vi "average m_error.vi"(1 "Num lights":dbl=2.0, 2 "Match error":waveform(dbl)[](array[waveform])) -> (0 "avg error":dbl[](array[numeric]))   [LabVIEW 2011]
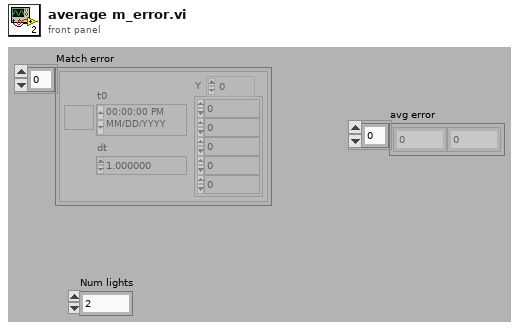
[diagram p1: front panel]
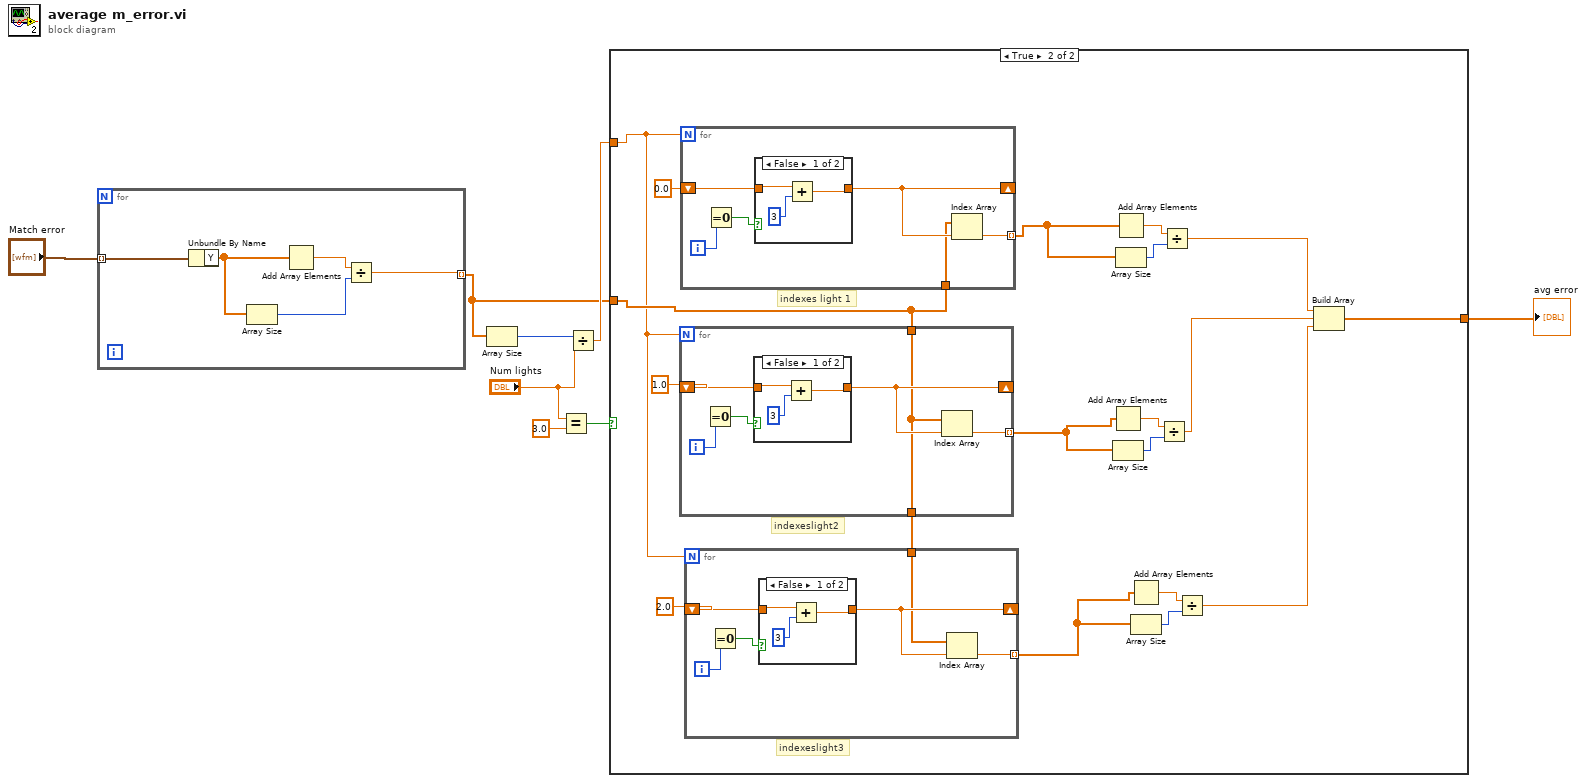
[diagram p0: block diagram]
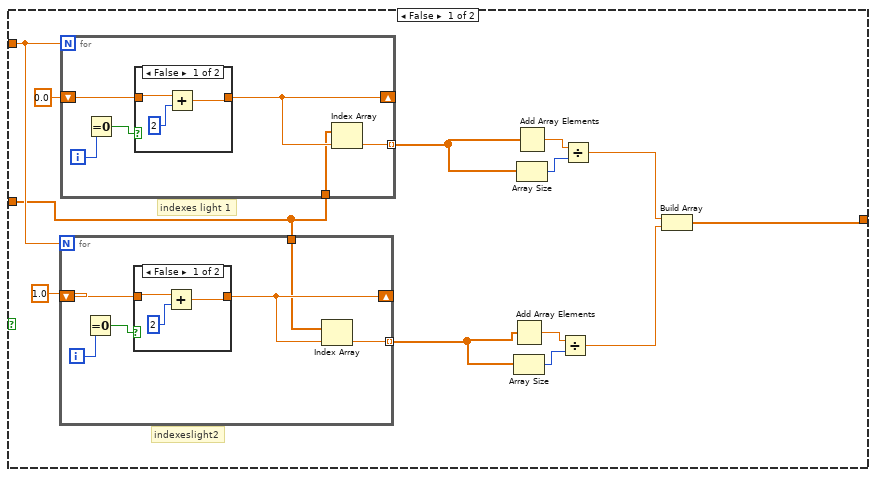
[diagram p2: hidden frame]
diagram:
  n1 = for {
    tunnel: "Match error" -> [w13] mode=indexing
    tunnel: [w9] -> w5 mode=indexing
    n2 = Unbundle By Name(w13) -> ("Y"=w12:dbl[])
    n3 = Array Size(array=w12) -> (size(s)=w10:i32)
    n4 = Add Array Elements(numeric array=w12) -> (sum=w11:dbl)
    n5 = Divide(x=w11, y=w10) -> (x/y=w9:dbl)
  }
  n6 = Array Size(array=w5) -> (size(s)=w7:i32)
  n7 = Equal?(x="Num lights", y=3.0) -> (x = y?=w2:bool)
  n8 = Divide(x=w7, y="Num lights") -> (x/y=w6:dbl)
  n9 = case shown="True" w2 {
    tunnel: w6 -> [w24 w60]
    tunnel: w5 -> [w23 w63]
    tunnel: [w14 w47] -> w1
    frame False {
      # "indexeslight2"
      # "indexes light 1"
      n10 = for {
        N: w24 -> [_]
        shift-right: [w29] -> _
        shift-left: 1.0 -> [w30]
        tunnel: [w28] -> w17 mode=indexing
        tunnel: w23 -> [w27]
        i -> [w32]
        n11 = Equal To 0?(x=w32) -> (x = 0?=w31:bool)
        n12 = case shown="False" w31 {
          tunnel: w30 -> [w35 w36]
          tunnel: [w33 w36] -> w29
          frame False {
            n13 = Add(x=w35, y=2) -> (x+y=w33:dbl)
          }
          frame True {
          }
        }
        n14 = Index Array(array=w27, index=w29) -> (element=w28:dbl)
      }
      n15 = for {
        N: w24 -> [_]
        shift-right: [w39] -> _
        shift-left: 0.0 -> [w40]
        tunnel: [w38] -> w18 mode=indexing
        tunnel: w23 -> [w37]
        i -> [w42]
        n16 = Equal To 0?(x=w42) -> (x = 0?=w41:bool)
        n17 = case shown="False" w41 {
          tunnel: w40 -> [w45 w46]
          tunnel: [w43 w46] -> w39
          frame False {
            n18 = Add(x=w45, y=2) -> (x+y=w43:dbl)
          }
          frame True {
          }
        }
        n19 = Index Array(array=w37, index=w39) -> (element=w38:dbl)
      }
      n20 = Add Array Elements(numeric array=w17) -> (sum=w20:dbl)
      n21 = Array Size(array=w17) -> (size(s)=w19:i32)
      n22 = Add Array Elements(numeric array=w18) -> (sum=w22:dbl)
      n23 = Array Size(array=w18) -> (size(s)=w21:i32)
      n24 = Divide(x=w20, y=w19) -> (x/y=w15:dbl)
      n25 = Divide(x=w22, y=w21) -> (x/y=w16:dbl)
      n26 = Build Array(w16, w15) -> (w14:dbl[])
    }
    frame True {
      # "indexeslight3"
      # "indexeslight2"
      # "indexes light 1"
      n27 = for {
        N: w60 -> [_]
        shift-right: [w78] -> _
        shift-left: 1.0 -> [w79]
        tunnel: [w77] -> w49 mode=indexing
        tunnel: w63 -> [w76]
        tunnel: [w76] -> w61
        i -> [w81]
        n28 = Equal To 0?(x=w81) -> (x = 0?=w80:bool)
        n29 = case shown="False" w80 {
          tunnel: w79 -> [w84 w85]
          tunnel: [w82 w85] -> w78
          frame False {
            n30 = Add(x=w84, y=3) -> (x+y=w82:dbl)
          }
          frame True {
          }
        }
        n31 = Index Array(array=w76, index=w78) -> (element=w77:dbl)
      }
      n32 = for {
        N: w60 -> [_]
        shift-right: [w88] -> _
        shift-left: 0.0 -> [w89]
        tunnel: [w87] -> w50 mode=indexing
        tunnel: w63 -> [w86]
        i -> [w91]
        n33 = Equal To 0?(x=w91) -> (x = 0?=w90:bool)
        n34 = case shown="False" w90 {
          tunnel: w89 -> [w94 w95]
          tunnel: [w92 w95] -> w88
          frame False {
            n35 = Add(x=w94, y=3) -> (x+y=w92:dbl)
          }
          frame True {
          }
        }
        n36 = Index Array(array=w86, index=w88) -> (element=w87:dbl)
      }
      n37 = for {
        N: w60 -> [_]
        shift-right: [w68] -> _
        shift-left: 2.0 -> [w69]
        tunnel: [w67] -> w48 mode=indexing
        tunnel: w61 -> [w66]
        i -> [w71]
        n38 = Equal To 0?(x=w71) -> (x = 0?=w70:bool)
        n39 = case shown="False" w70 {
          tunnel: w69 -> [w74 w75]
          tunnel: [w72 w75] -> w68
          frame False {
            n40 = Add(x=w74, y=3) -> (x+y=w72:dbl)
          }
          frame True {
          }
        }
        n41 = Index Array(array=w66, index=w68) -> (element=w67:dbl)
      }
      n42 = Add Array Elements(numeric array=w49) -> (sum=w57:dbl)
      n43 = Array Size(array=w49) -> (size(s)=w56:i32)
      n44 = Add Array Elements(numeric array=w50) -> (sum=w59:dbl)
      n45 = Array Size(array=w50) -> (size(s)=w58:i32)
      n46 = Add Array Elements(numeric array=w48) -> (sum=w55:dbl)
      n47 = Array Size(array=w48) -> (size(s)=w54:i32)
      n48 = Divide(x=w57, y=w56) -> (x/y=w52:dbl)
      n49 = Divide(x=w59, y=w58) -> (x/y=w53:dbl)
      n50 = Divide(x=w55, y=w54) -> (x/y=w51:dbl)
      n51 = Build Array(w53, w52, w51) -> (w47:dbl[])
    }
  }
  "avg error" <- w1
